vi "Data Type Valid.vi"(8 "error in":errorcluster, 10 "Valid":bool, 11 "Error Msg":string) -> (0 "error out":errorcluster)   [LabVIEW 2020, in "Data Type Scripting.lvlib"]
doc: "_____\nCreated using DQMH Event Scripter 6.0.0.122."
uses:
  Data Type Scripting.lvlib
  Data Type Valid Argument--cluster.ctl
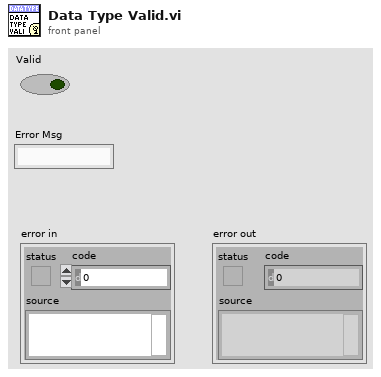
[diagram p1: front panel]
types:
  T1 = typedef "Data Type Scripting.lvlib/Data Type Valid Argument--cluster.ctl" = cluster{"Valid":bool, "Error Msg":string}
  T2 = typedef "Data Type Scripting.lvlib/Broadcast Events--cluster.ctl" = cluster{"Module Did Init":refnum<user-event>, "Status Updated":refnum<user-event>, "Error Reported":refnum<user-event>, "Module Did Stop":refnum<user-event>, "Update Module Execution Status":refnum<user-event>, "Template Path":refnum<user-event>, "Poly List":refnum<user-event>, "Poly Details":refnum<user-event>, "Data Type Valid":refnum<user-event>}
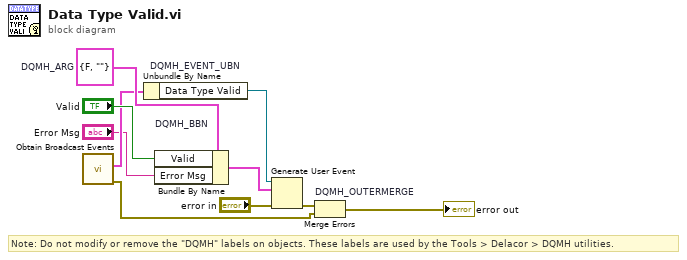
[diagram p0: block diagram]
diagram:
  w5 = T1 {"Valid"=FALSE, "Error Msg"=""}  # DQMH_ARG
  # "Note: Do not modify or remove the \"DQMH\" labels on objects. These labels are used by the Tools > Delacor > DQMH utilities."
  n1 = call "Obtain Broadcast Events.vi"() -> ("error out"=w3:errorcluster, "Data Type Scripting Broadcast Events"=w2:T2)  [unwired: 10 in]
  n2 = Unbundle By Name "DQMH_EVENT_UBN"(w2) -> ("Data Type Valid"=w7:refnum<user-event>)
  n3 = Bundle By Name "DQMH_BBN"(cluster=w5, "Valid"="Valid", "Error Msg"="Error Msg") -> (w8:T1)
  n4 = Generate User Event(user event=w7, event data cluster=w8, error in="error in") -> (error out=w6:errorcluster)  [unwired: 1 in, 1 out]
  n5 = Merge Errors "DQMH_OUTERMERGE"(w6, w3) -> (→"error out":errorcluster)
